vi "MisurazioniString.vi"(8 "error in (no error)":errorcluster, 10 "index":i32, 11 "Calibration data":T1 {"controls"."umidita" format="%.1g"; "controls"."temperatura_c" format="%.1g"; "controls"."incertezza" format="%.1g"; "controls"."deviazione_standard" format="%.1g"; "controls"."mpe_min" format="%.1g"; "controls"."mpe_max" format="%.1g"; "controls"."riferimento_obiettivo" format="%.1g"}) -> (0 "error out":errorcluster, 2 "index":i32, 3 "String":string)   [LabVIEW 2019]
uses:
  ByteGSAPIBase/CalibrationMeasurements/BodyCalibrazioneMisure.ctl
  ByteGSAPIBase/ByteGSAPIBase.lvclass
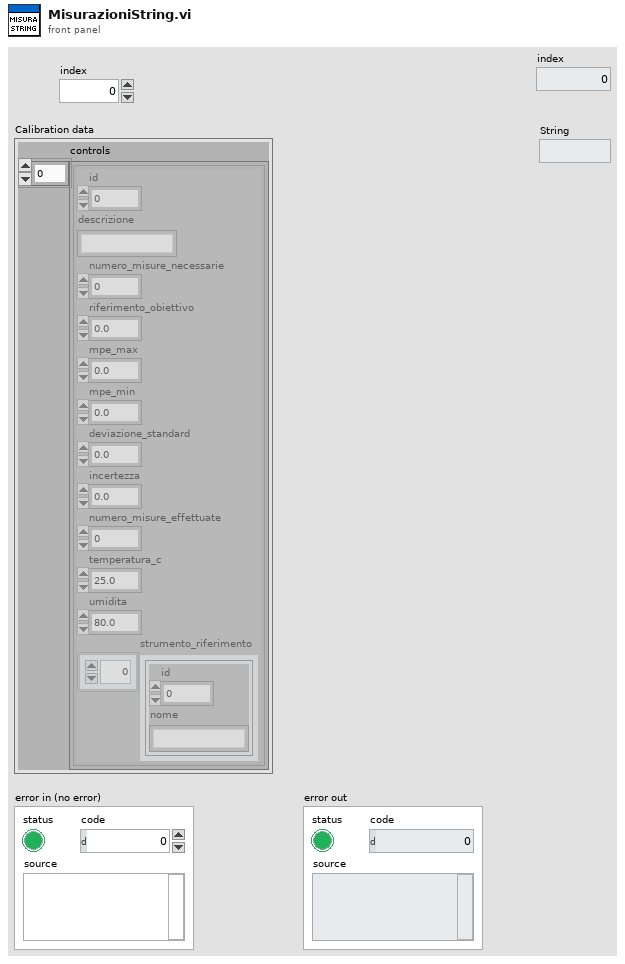
[diagram p1: front panel]
types:
  T1 = typedef "ByteGSWebAPI.lvlib/ByteGSAPIBase.lvclass/BodyCalibrazioneMisure.ctl" = cluster{"controls":cluster{"id":u16, "descrizione":string, "numero_misure_necessarie":u16, "riferimento_obiettivo":dbl, "mpe_max":dbl, "mpe_min":dbl, "deviazione_standard":dbl, "incertezza":dbl, "numero_misure_effettuate":u32, "temperatura_c":dbl, "umidita":dbl, "strumento_riferimento":cluster{"id":u16, "nome":string}[]}[]}
  T2 = cluster{"id":u16, "descrizione":string, "numero_misure_necessarie":u16, "riferimento_obiettivo":dbl, "mpe_max":dbl, "mpe_min":dbl, "deviazione_standard":dbl, "incertezza":dbl, "numero_misure_effettuate":u32, "temperatura_c":dbl, "umidita":dbl, "strumento_riferimento":cluster{"id":u16, "nome":string}[]}[]
  T3 = cluster{"id":u16, "descrizione":string, "numero_misure_necessarie":u16, "riferimento_obiettivo":dbl, "mpe_max":dbl, "mpe_min":dbl, "deviazione_standard":dbl, "incertezza":dbl, "numero_misure_effettuate":u32, "temperatura_c":dbl, "umidita":dbl, "strumento_riferimento":cluster{"id":u16, "nome":string}[]}
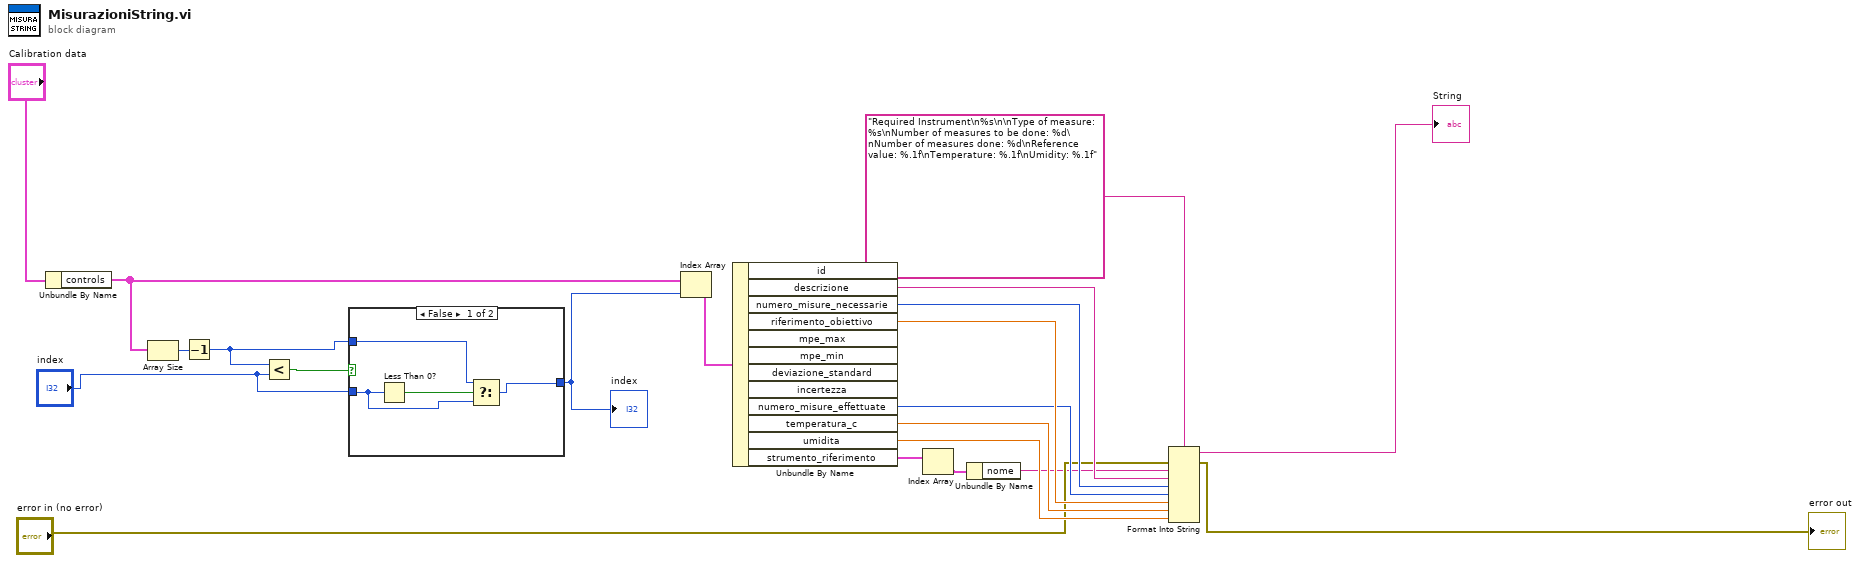
[diagram p0: block diagram]
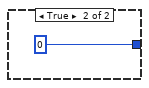
[diagram p2: hidden frame]
diagram:
  n1 = Unbundle By Name("Calibration data") -> ("controls"=w4:T2)
  n2 = Array Size(array=w4) -> (size(s)=w2:i32)
  n3 = Decrement(x=w2) -> (x-1=w1:i32)
  n4 = Less?(x=w1, y="index") -> (x < y?=w6:bool)
  n5 = case shown="False" w6 {
    tunnel: [w23 0] -> w5
    tunnel: "index" -> [w24 _]
    tunnel: w1 -> [w22 _]
    frame False {
      n6 = Less Than 0?(x=w24) -> (x < 0?=w25:bool)
      n7 = Select(t=w22, s=w25, f=w24) -> (s? t:f=w23:i32)
    }
    frame True {
    }
  }
  "index" <- w5
  n8 = Index Array(array=w4, index=w5) -> (element=w8:T3)
  n9 = Unbundle By Name(w8) -> ("descrizione"=w15:string, "numero_misure_necessarie"=w16:u16, "riferimento_obiettivo"=w18:dbl, "numero_misure_effettuate"=w17:u32, "temperatura_c"=w19:dbl, "umidita"=w20:dbl, "strumento_riferimento"=w9:cluster{"id":u16, "nome":string}[])  [unwired: 5 out]
  n10 = Index Array(array=w9) -> (element=w10:cluster{"id":u16, "nome":string})  [unwired: 1 in]
  n11 = Unbundle By Name(w10) -> ("nome"=w11:string)
  n12 = Format Into String(format string="Required Instrument\n%s\n\nType of measure: %s\nNumber of measures to be done: %d\nNumber of measures done: %d\nReference value: %.1f\nTemperature: %.1f\nUmidity: %.1f", error in="error in (no error)", w11, w15, w16, w17, w18, w19, w20) -> (resulting string=→"String":string, error out=→"error out":errorcluster)  [unwired: 1 in]
